vi "Logic_Close_Connection.vi"(4 "error in (no error)":errorcluster, 7 "Session Ref In":T1) -> (0 "error out":errorcluster, 3 "Python Session Out":refnum<k35>)   [LabVIEW 2023]
doc: "Close the connection to the Saleae Logic2 software."
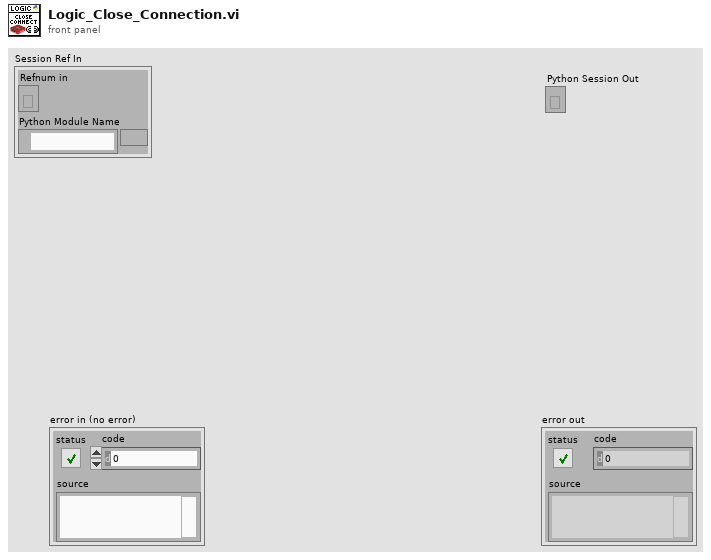
[diagram p1: front panel]
types:
  T1 = cluster{"Refnum in":refnum<k35>, "Python Module Name":path}
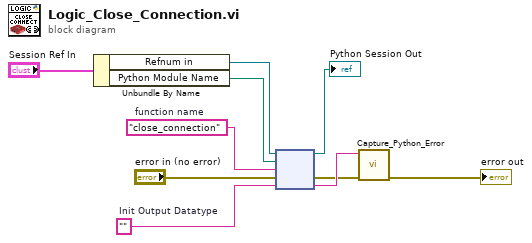
[diagram p0: block diagram]
diagram:
  w9 = "close_connection"  # function name
  w8 = ""  # Init Output Datatype
  n1 = Unbundle By Name("Session Ref In") -> ("Refnum in"=w6:refnum<k35>, "Python Module Name"=w5:path)
  n2 = node(w6, w5, w9, "error in (no error)", w8) -> (→"Python Session Out":refnum<k35>, w2:errorcluster, w3:string)  [unwired: 2 out]
  n3 = call "Capture_Python_Error.vi"("error in (no error)"=w2, "Error Message (start with ERROR)"=w3) -> ("error out"=→"error out":errorcluster)  [unwired: 9 in]
